vi "iterate func (SubVI).vi"(11 "int i; Ref":refnum<vi>) -> (3 "Actual Value (i)":i32)   [LabVIEW 2017]
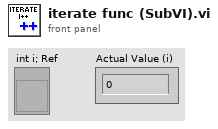
[diagram p1: front panel]
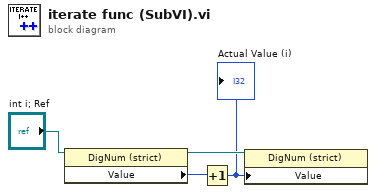
[diagram p0: block diagram]
diagram:
  n1 = property class="DigNum (strict)"(reference="int i; Ref") -> (reference out=w3:refnum<vi>, "Value"=w4:i32)  [unwired: 1 in, 1 out]
  n2 = Increment(x=w4) -> (x+1=w1:i32)
  "Actual Value (i)" <- w1
  n3 = property class="DigNum (strict)"(reference=w3, "Value"=w1) -> ()  [unwired: 1 in, 2 out]
